vi "Easy Print VI Panel or Documentation (refnum).vi"(6 "custom contents options":T14 {"list of controls options"."list which controls?" items=["all controls", "connected controls"]}, 7 "layout options":T2={"orientation (unchanged)"=0, "panel scaling for page (unchanged)"=0, "margins"={"override VI margins (false)"=FALSE, "margins (1.00)"={"top"=1.0, "left"=1.0, "right"=1.0, "bottom"=1.0}, "measurement system (default)"=0}, "printer options"={"destination printer name (current)"="", "printing method (unchanged)"=0, "color or monochrome (unchanged)"=0}, "page header options"={"page headers (unchanged)"=0, "page header content options"={"Include VI Name"=TRUE, "Include VI Path"=TRUE, "Include Last Modification Date"=TRUE, "Include Date Printed"=TRUE, "Include Page Number"=TRUE, "Include VI Icon"=TRUE}}} {"page header options"."page headers (unchanged)" items=["Unchanged", "Include page headers", "Do not include page headers"]; "printer options"."color or monochrome (unchanged)" items=["Unchanged", "Color/grayscale", "Monochrome"]; "printer options"."printing method (unchanged)" items=["Unchanged", "Standard", "PostScript", "Bitmap"]; "panel scaling for page (unchanged)" items=["Unchanged", "No Scaling", "Scale front panel to fit"]; "orientation (unchanged)" items=["Unchanged", "portrait", "landscape"]; "margins"."measurement system (default)" items=["Default", "US", "Metric"]; "margins"."margins (1.00)"."right" format="%.2f"; "margins"."margins (1.00)"."bottom" format="%.2f"; "margins"."margins (1.00)"."top" format="%.2f"; "margins"."margins (1.00)"."left" format="%.2f"}, 8 "error in (no error)":errorcluster, 9 "report type (Quick Print)":T1 items=["Quick Print", "Standard Report", "HTML", "Word", "Excel"], 10 "contents (complete front panel)":T16 items=["Complete front panel", "Visible portion of front panel", "Icon, description, panel and diagram", "Documentation: Using the panel", "Documentation: Using as a subVI", "Documentation: Complete", "Documentation: Custom"], 11 "VI reference":refnum<vi>) -> (0 "error out":errorcluster, 3 "report out":refnum<class "NI_report.lvclass">)   [LabVIEW 2017, in "NI_ReportGenerationCore.lvlib"]
doc: "Prints a front panel or VI documentation or saves the front panel or VI documentation to a report. Wire data to the <B>VI path</B> input to determine the polymorphic instance to use or manually select the instance."
uses:
  <vilib>/Utility/NIReport.llb/NI_ReportGenerationCore.lvlib
  <vilib>/printing/EasyPrintingControls.llb/contents.ctl
  <vilib>/printing/EasyPrintingControls.llb/layout_options.ctl
  <vilib>/printing/EasyPrintingControls.llb/orientation.ctl
  <vilib>/printing/EasyPrintingControls.llb/panel_scaling_for_page.ctl
  <vilib>/printing/EasyPrintingControls.llb/margins.ctl
  <vilib>/printing/EasyPrintingControls.llb/margin_values.ctl
  <vilib>/printing/EasyPrintingControls.llb/measurement_system.ctl
  <vilib>/printing/EasyPrintingControls.llb/printer_options.ctl
  <vilib>/printing/EasyPrintingControls.llb/printing_method.ctl
  <vilib>/printing/EasyPrintingControls.llb/color_or_monochrome.ctl
  <vilib>/printing/EasyPrintingControls.llb/page_header_options.ctl
  <vilib>/printing/EasyPrintingControls.llb/page_headers.ctl
  <vilib>/printing/EasyPrintingControls.llb/page_header_content_options.ctl
  <vilib>/printing/EasyPrintingControls.llb/custom_contents_options.ctl
  <vilib>/printing/EasyPrintingControls.llb/list_which_controls.ctl
  <vilib>/Utility/NIReport.llb/NI_report.lvclass
  <vilib>/printing/EasyPrintingControls.llb/report_type.ctl
  <vilib>/printing/EasyPrintingControls.llb/report_type_ENUM.ctl
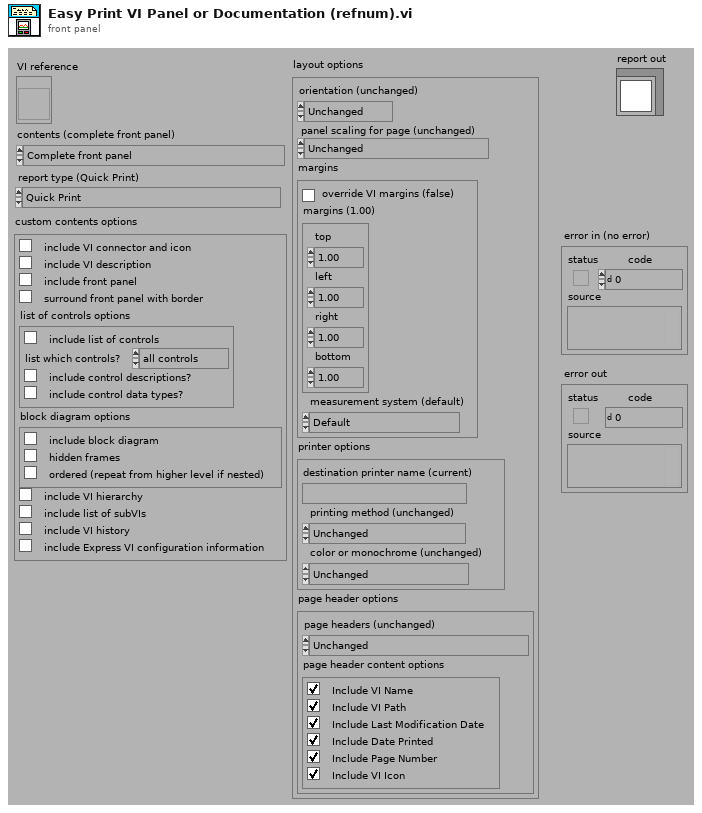
[diagram p1: front panel]
types:
  T1 = typedef "NI_ReportGenerationCore.lvlib/report_type.ctl" = u16
  T2 = typedef "NI_ReportGenerationCore.lvlib/layout_options.ctl" = cluster{"orientation (unchanged)":T3, "panel scaling for page (unchanged)":T4, "margins":T5, "printer options":T8, "page header options":T11}
  T3 = typedef "NI_ReportGenerationCore.lvlib/orientation.ctl" = u16
  T4 = typedef "NI_ReportGenerationCore.lvlib/panel_scaling_for_page.ctl" = u16
  T5 = typedef "NI_ReportGenerationCore.lvlib/margins.ctl" = cluster{"override VI margins (false)":bool, "margins (1.00)":T6, "measurement system (default)":T7}
  T6 = typedef "NI_ReportGenerationCore.lvlib/margin_values.ctl" = cluster{"top":dbl, "left":dbl, "right":dbl, "bottom":dbl}
  T7 = typedef "NI_ReportGenerationCore.lvlib/measurement_system.ctl" = u16
  T8 = typedef "NI_ReportGenerationCore.lvlib/printer_options.ctl" = cluster{"destination printer name (current)":string, "printing method (unchanged)":T9, "color or monochrome (unchanged)":T10}
  T9 = typedef "NI_ReportGenerationCore.lvlib/printing_method.ctl" = u16
  T10 = typedef "NI_ReportGenerationCore.lvlib/color_or_monochrome.ctl" = u16
  T11 = typedef "NI_ReportGenerationCore.lvlib/page_header_options.ctl" = cluster{"page headers (unchanged)":T12, "page header content options":T13}
  T12 = typedef "NI_ReportGenerationCore.lvlib/page_headers.ctl" = u16
  T13 = typedef "NI_ReportGenerationCore.lvlib/page_header_content_options.ctl" = cluster{"Include VI Name":bool, "Include VI Path":bool, "Include Last Modification Date":bool, "Include Date Printed":bool, "Include Page Number":bool, "Include VI Icon":bool}
  T14 = typedef "NI_ReportGenerationCore.lvlib/custom_contents_options.ctl" = cluster{"include VI connector and icon":bool, "include VI description":bool, "include front panel":bool, "surround front panel with border":bool, "list of controls options":cluster{"include list of controls":bool, "list which controls?":T15, "include control descriptions?":bool, "include control data types?":bool}, "block diagram options":cluster{"include block diagram":bool, "hidden frames":bool, "ordered (repeat from higher level if nested)":bool}, "include VI hierarchy":bool, "include list of subVIs":bool, "include VI history":bool, "include Express VI configuration information":bool}
  T15 = typedef "NI_ReportGenerationCore.lvlib/list_which_controls.ctl" = u16
  T16 = typedef "NI_ReportGenerationCore.lvlib/contents.ctl" = u16
  T17 = typedef "NI_ReportGenerationCore.lvlib/report_type_ENUM.ctl" = enum16{"Quick Print", "Standard Report", "HTML", "Word", "Excel"}
  T18 = enum16{"Standard Report", "HTML", "Word", "Excel"}
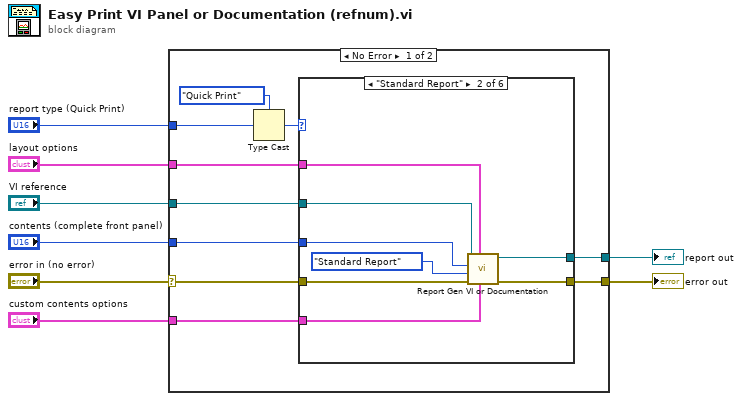
[diagram p0: block diagram]
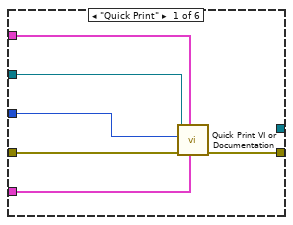
[diagram p2: hidden frame]
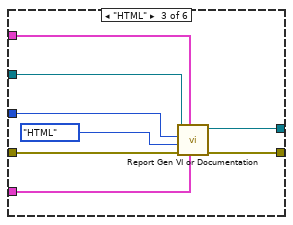
[diagram p3: hidden frame]
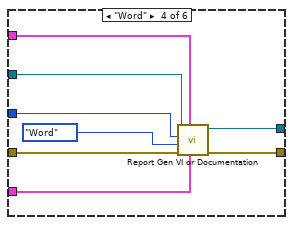
[diagram p4: hidden frame]
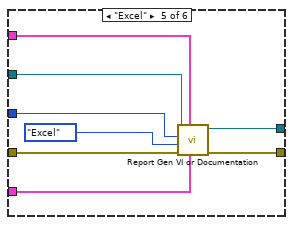
[diagram p5: hidden frame]
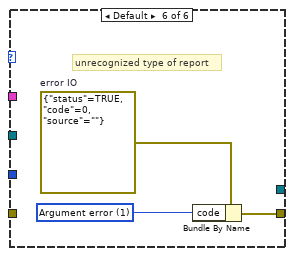
[diagram p6: hidden frame]
diagram:
  n1 = case shown="No Error" "error in (no error)" {
    selector: "error in (no error)" -> [w16 w60]
    tunnel: [w17 w60] -> w7
    tunnel: [w15 _] -> w6
    tunnel: "layout options" -> [w13 _]
    tunnel: "VI reference" -> [w12 _]
    tunnel: "report type (Quick Print)" -> [w11 _]
    tunnel: "contents (complete front panel)" -> [w10 _]
    tunnel: "custom contents options" -> [w9 _]
    frame No Error {
      n2 = Type Cast(type=report_type_ENUM."Quick Print" ("report type ENUM"), x=w11) -> (*(type *) &x=w18:T17)
      n3 = case shown="\"Standard Report\"" w18 {
        tunnel: [w23 w26 w34 w42 w50 w57] -> w17
        tunnel: w12 -> [w19 w25 w33 w41 w49 _]
        tunnel: w10 -> [w22 w31 w39 w46 w54 _]
        tunnel: w13 -> [w21 w32 w40 w47 w55 _]
        tunnel: w9 -> [w20 w29 w37 w44 w52 _]
        tunnel: w16 -> [w24 w30 w38 w45 w51 _]
        tunnel: [_ w28 w36 w48 w56 _] -> w15
        frame "Quick Print" {
          n4 = call <vilib>:"Quick Print VI or Documentation.vi"("custom contents options"=w20, "layout options"=w21, "error in (no error)"=w24, "contents (complete front panel)"=w22, "VI reference"=w19) -> ("error out"=w23:errorcluster)  [unwired: 6 in]
        }
        frame "Standard Report" {
          n5 = call <vilib>:"Report Gen VI or Documentation.vi"("custom contents options"=w29, "layout options"=w32, "error in (no error)"=w30, "report type"=T18."Standard Report", "contents (complete front panel)"=w31, "VI reference"=w25) -> ("error out"=w26:errorcluster, "report out"=w28:refnum<class "NI_report.lvclass">)  [unwired: 4 in]
        }
        frame "HTML" {
          n6 = call <vilib>:"Report Gen VI or Documentation.vi"("custom contents options"=w37, "layout options"=w40, "error in (no error)"=w38, "report type"=T18."HTML", "contents (complete front panel)"=w39, "VI reference"=w33) -> ("error out"=w34:errorcluster, "report out"=w36:refnum<class "NI_report.lvclass">)  [unwired: 4 in]
        }
        frame "Word" {
          n7 = call <vilib>:"Report Gen VI or Documentation.vi"("custom contents options"=w44, "layout options"=w47, "error in (no error)"=w45, "report type"=T18."Word", "contents (complete front panel)"=w46, "VI reference"=w41) -> ("error out"=w42:errorcluster, "report out"=w48:refnum<class "NI_report.lvclass">)  [unwired: 4 in]
        }
        frame "Excel" {
          n8 = call <vilib>:"Report Gen VI or Documentation.vi"("custom contents options"=w52, "layout options"=w55, "error in (no error)"=w51, "report type"=T18."Excel", "contents (complete front panel)"=w54, "VI reference"=w49) -> ("error out"=w50:errorcluster, "report out"=w56:refnum<class "NI_report.lvclass">)  [unwired: 4 in]
        }
        frame Default {
          w59 = errorcluster {"status"=TRUE, "code"=0, "source"=""}  # error IO
          w58 = 1 items=["No error", "Argument error", "Memory is full", "Out of zone", "End of file", "File already open", "Generic file I/O error", "File not found", "File permission error", "Disk is full", "Duplicate path", "Too many files open", "System feature not enabled", "Resource file not found", "Cannot add resource", "Resource not found", "Image not found", "Image memory error", "Pen does not exist", "Config type invalid", "Config token not found", "Config parse error", "Config memory error", "Bad external code format", "Bad external code offset", "External code not present", "Null window", "Destroy window error", "Null menu", "Print aborted", "Bad print record", "Print driver error", "Windows error during printing", "Memory error during printing", "Print dialog error", "Generic print error", "Invalid device refnum", "Device not found", "Device parameter error", "Device unit error", "Cannot open device", "Device call aborted", "Generic error", "Cancelled by user", "Object ID too low", "Object ID too high", "Object not in heap", "Unknown heap", "Unknown object (invalid DefProc)", "Unknown object (DefProc not in table)", "Message out of range", "Invalid (null) method", "Unknown message", "Manager call not supported", "Bad address", "Network operation in progress", "Network operation timed out", "Connection is busy", "Network attribute not supported", "Network error", "Address in use", "System out of memory", "Connection aborted", "Connection refused", "Not connected", "Already connected", "Connection closed", "Initialization error (interapplication manager)", "Bad occurrence", "Wait on unbound occurrence handler", "Occurrence queue overflow", "Datalog type conflict", "Unused", "Unrecognized type (interapplication manager)", "Memory corrupt", "Failed to make temporary DLL", "Old CIN version", "Drag socket not found", "Failed to load drop-object", "Failed to register OLE object", "Failed to release OLE object", "Format specifier type mismatch", "Unknown format specifier", "Too few format specifiers", "Too many format specifiers", "Scan failed", "Newer CIN version", "Error converting to variant", "Runtime menu error", "Password tampered", "Variant attribute not found", "Incompatible variant data type", "Event data is not available", "Event Store is not present", "Occurrence is not found", "Event Queue is not created", "Event info is not available", "Refnum passed is NULL", "Error retrieving Class GUID", "Error retrieving CoClass GUID", "Error retrieving TypeLib GUID.", "Bad built application magic bytes.", "Specific driver is different from the specific driver associated with the Logical Name.", "There is no session opened to the class driver.", "Max Error", "MAX - Error with config objects", "MAX - Error loading configuration", "MAX - Group not supported"]
          # "unrecognized type of report"
          n9 = Bundle By Name(cluster=w59, "code"=w58) -> (w57:errorcluster)
        }
      }
    }
    frame Error {
    }
  }
  "error out" <- w7
  "report out" <- w6
